vi "Snare_Brush.vi"(10 "M":fxp<+,32,32>, 11 "Trigger":bool) -> (3 "Brushes Out":fxp<+/-,8,8>)   [LabVIEW 2015]
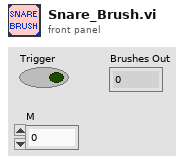
[diagram p1: front panel]
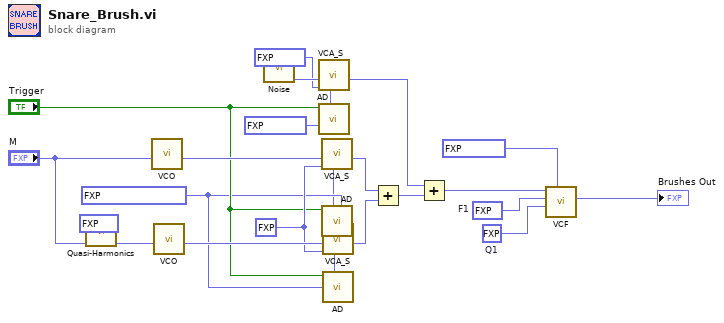
[diagram p0: block diagram]
diagram:
  w8 = fxp<+,8,0> 0.5 ("Amount 2")
  w3 = fxp<+,16,0> 0.000213623046875 ("1/Decay 2")
  w19 = fxp<+/-,18,18> 1.0  # Q1
  w18 = fxp<+/-,18,18> 3700.0  # F1
  n1 = call "Quasi-Harmonics.vi"("Relative Freq"=fxp<+,8,3> 1.3125 ("relative f 2"), "1st partial"="M") -> ("Result Partial"=w11:fxp<+,32,32>)  [unwired: 9 in]
  n2 = call "VCO.vi"("M"="M") -> ("Sine Sample"=w21:fxp<+/-,8,8>)  [unwired: 10 in]
  n3 = call "VCO.vi"("M"=w11) -> ("Sine Sample"=w22:fxp<+/-,8,8>)  [unwired: 10 in]
  n4 = call "Noise.vi"() -> ("White Noise Out"=w16:fxp<+/-,8,8>)  [unwired: 11 in]
  n5 = call "AD.vi"("1/Decay"=fxp<+,16,0> 7.62939453125e-05 ("Noise 1/D"), "Trigger"="Trigger") -> ("Sample Out"=w5:fxp<+,8,0>)  [unwired: 9 in]
  n6 = call "VCA_S.vi"("EG"=w5, "Amount"=fxp<+,8,0> 0.88671875 ("Noise Amount"), "Sample In"=w16) -> ("Sample Out"=w10:fxp<+/-,8,8>)  [unwired: 8 in]
  n7 = call "AD.vi"("1/Decay"=w3, "Trigger"="Trigger") -> ("Sample Out"=w2:fxp<+,8,0>)  [unwired: 9 in]
  n8 = call "VCA_S.vi"("EG"=w2, "Amount"=w8, "Sample In"=w21) -> ("Sample Out"=w13:fxp<+/-,8,8>)  [unwired: 8 in]
  n9 = call "AD.vi"("1/Decay"=w3, "Trigger"="Trigger") -> ("Sample Out"=w1:fxp<+,8,0>)  [unwired: 9 in]
  n10 = call "VCA_S.vi"("EG"=w1, "Amount"=w8, "Sample In"=w22) -> ("Sample Out"=w14:fxp<+/-,8,8>)  [unwired: 8 in]
  n11 = Add(x=w13, y=w14) -> (x+y=w15:fxp<+/-,8,8>)
  n12 = Add(x=w10, y=w15) -> (x+y=w17:fxp<+/-,8,8>)
  n13 = call "VCF.vi"("Amount"=fxp<+,8,0> 0.99609375, "Q1"=w19, "F1"=w18, "Sample In"=w17) -> ("LP Out"=→"Brushes Out":fxp<+/-,8,8>)  [unwired: 5 in, 2 out]
